vi "Manage Collision.vi"(11 "Ball-Goal Post in":refnum<class "Ball-Goal Post.lvclass">) -> (1 "Remove GB Components out":refnum<class "Game Board Component.lvclass">[](array[class]), 2 "GB Components out":refnum<class "Game Board Component.lvclass">[](array[class]))   [LabVIEW 2024, in "Ball-Goal Post.lvclass"]
doc: "MIT Licence\nCopyright (c) 2024 David Grollier"
uses:
  Ball-Goal Post.lvclass
  Game Componants/Game Board Component/Game Board Component.lvclass
  Game Componants/Game Board Component/Fixed/Board/Goal post/Goal Post.lvclass
  Collision.lvclass/Collision.ctl
  Game Componants/Game Board Component/Movable/Movable.lvclass/Movable.ctl
  Game Componants/Game Componants.lvclass/Game Componants.ctl
  Game Componants/Game Board Component/Movable/Movable.lvclass
  Game Componants/Game Board/Game Board.lvclass
  Game Componants/Game Componants.lvclass
  Collision.lvclass
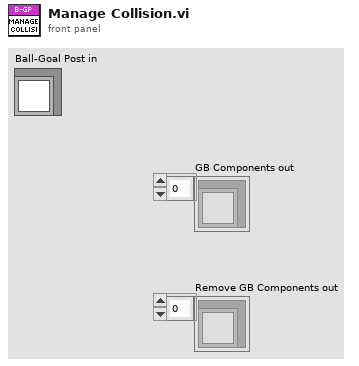
[diagram p1: front panel]
types:
  T1 = typedef "Velocity.ctl" = cluster{"Vx":dbl, "Vy":dbl}
  T2 = typedef "Coordinates.ctl" = cluster{"x":dbl, "y":dbl}
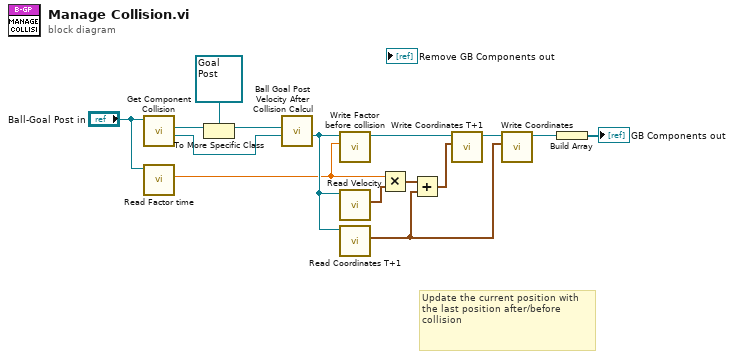
[diagram p0: block diagram]
diagram:
  # "Update the current position with the last position after/before collision"
  n1 = call "Get Component Collision.vi"("Collision in"="Ball-Goal Post in") -> ("Movable out"=w12:refnum<class "Movable.lvclass">, "GB Component out"=w13:refnum<class "Game Board Component.lvclass">)  [unwired: 9 in]
  n2 = call "Read Factor time.vi"("Collision in"="Ball-Goal Post in") -> ("Factor time"=w1:dbl)  [unwired: 10 in]
  n3 = To More Specific Class(target class=refnum<class "Goal Post.lvclass"> refnum ("Goal post in"), reference=w13) -> (specific class reference=w14:refnum<class "Goal Post.lvclass">)  [unwired: 1 in, 1 out]
  n4 = call "Ball Goal Post Velocity After Collision Calcul.vi"("Movable in"=w12, "Goal post in"=w14) -> ("Movable out"=w4:refnum<class "Movable.lvclass">)  [unwired: 9 in]
  n5 = call "Write Factor before collision.vi"("Factor before collision"=w1, "Movable in"=w4) -> ("Movable out"=w2:refnum<class "Movable.lvclass">)  [unwired: 9 in]
  n6 = call-dynamic "Read Velocity.vi"("Movable in"=w4) -> ("Velocity"=w10:T1)  [unwired: 10 in]
  n7 = call "Read Coordinates T+1.vi"("Movable in"=w4) -> ("Coordinates"=w6:T2)  [unwired: 10 in]
  n8 = Multiply(x=w1, y=w10) -> (x*y=w11:T1)
  n9 = Add(x=w11, y=w6) -> (x+y=w8:T1)
  n10 = call "Write Coordinates T+1.vi"("Coordinates"=w8, "Movable in"=w2) -> ("Movable out"=w7:refnum<class "Movable.lvclass">)  [unwired: 9 in]
  n11 = call "Write Coordinates.vi"("Coordinates"=w6, "Game Componants in"=w7) -> ("Game Componants out"=w5:refnum<class "Movable.lvclass">)  [unwired: 9 in]
  n12 = Build Array(w5) -> (→"GB Components out":refnum<class "Movable.lvclass">[])
